vi "Actor Core.vi"(8 "error in":errorcluster, 11 "Settings View in":refnum<class "Settings View.lvclass">) -> (0 "error out":errorcluster={"status"=TRUE, "code"=1556, "source"="In Place Element Structure in Actor Framework.lvlib:Message Priority Queue.lvclass:Priority Enqueue.vi:2960001->Actor Framework MVC.lvlib:Abstract View.lvlib:Abstract View.lvclass:Actor Core.vi:5880008->Settings View.lvlib:Settings View.lvclass:Actor Core.vi"}, 3 "Actor out":refnum<class "Actor.lvclass">)   [LabVIEW 2020, in "Settings View.lvlib" / "Settings View.lvclass"]
doc: "(<B>Filename</B>: Actor Framework.lvlib:Actor.lvclass:Actor Core.vi)\n\nReceives messages to the actor, reacts to them, and initiates any error handling that may shut the actor down.\n\nDescendant classes may override this VI to append parallel tasks for the actor to complete while it handles messages. Overrides use the Call Parent Method node."
uses:
  Settings View.lvclass
  C:/Program Files/National Instruments/LabVIEW 2020/vi.lib/ActorFramework/Actor/Actor.lvclass
  <vilib>/ActorFramework/Actor/Actor.lvclass
  <vilib>/ActorFramework/Actor/Actor.lvclass/Actor.ctl
  <vilib>/ActorFramework/Message Enqueuer/Message Enqueuer.lvclass/Message Enqueuer.ctl
  Settings View Messages/Broadcast Show Grid Msg/Broadcast Show Grid Msg.lvclass/Broadcast Show Grid Msg.ctl
  Settings View Messages/Broadcast Show Origin Msg/Broadcast Show Origin Msg.lvclass/Broadcast Show Origin Msg.ctl
  Settings View Messages/Broadcast Show Tool Label Msg/Broadcast Show Tool Label Msg.lvclass/Broadcast Show Tool Label Msg.ctl
  Settings View Messages/Broadcast Brush Width Msg/Broadcast Brush Width Msg.lvclass/Broadcast Brush Width Msg.ctl
  Settings View Messages/Broadcast Color Table Msg/Broadcast Color Table Msg.lvclass/Broadcast Color Table Msg.ctl
  <vilib>/ActorFramework/Message Enqueuer/Init from Existing Queue.vi
  <vilib>/ActorFramework/Message Enqueuer/Enqueue.vi
  Settings View Messages/Broadcast Show Grid Msg/Broadcast Show Grid Msg.lvclass
  C:/Program Files/National Instruments/LabVIEW 2020/vi.lib/ActorFramework/Message/Message.lvclass
  Settings View Messages/Broadcast Show Origin Msg/Broadcast Show Origin Msg.lvclass
  Settings View Messages/Broadcast Show Tool Label Msg/Broadcast Show Tool Label Msg.lvclass
  Settings View Messages/Broadcast Brush Width Msg/Broadcast Brush Width Msg.lvclass
  Settings View Messages/Broadcast Color Table Msg/Broadcast Color Table Msg.lvclass
  Controllers/UI Controller/UI Controller Messages/Initialize Main View Msg/Initialize Main View Msg.lvclass
  Controllers/UI Controller/UI Controller Messages/Update Occupied Area Msg/Update Occupied Area Msg.lvclass
  <vilib>/ActorFramework/Message Priority Queue/Priority Enqueue.vi
  <vilib>/ActorFrameworkMVC/Abstract View/Abstract View/Abstract View.lvclass
  <vilib>/ActorFramework/Message Enqueuer/Message Enqueuer.lvclass
panel:
  in  "Color Table":T1={"Occupied Color"={"Value"=0, "Color"=0}, "Free Color"={"Value"=254, "Color"=13421772}, "Unknown Color"={"Value"=205, "Color"=16777215}}
  in  "Set Button":bool
  in  "Brush Width Slider":i32(slide)=3 scale=1.0..10.0
  in  "Show Tool Label Button":bool=TRUE
  in  "Show Origin Button":bool
  in  "Show Grid Button":bool
  # "Show grid"
  # "Show origin"
  # "Show tool label"
  # "Brush width"
  # "Occupied color"
  # "Free color"
  # "Unknown color"
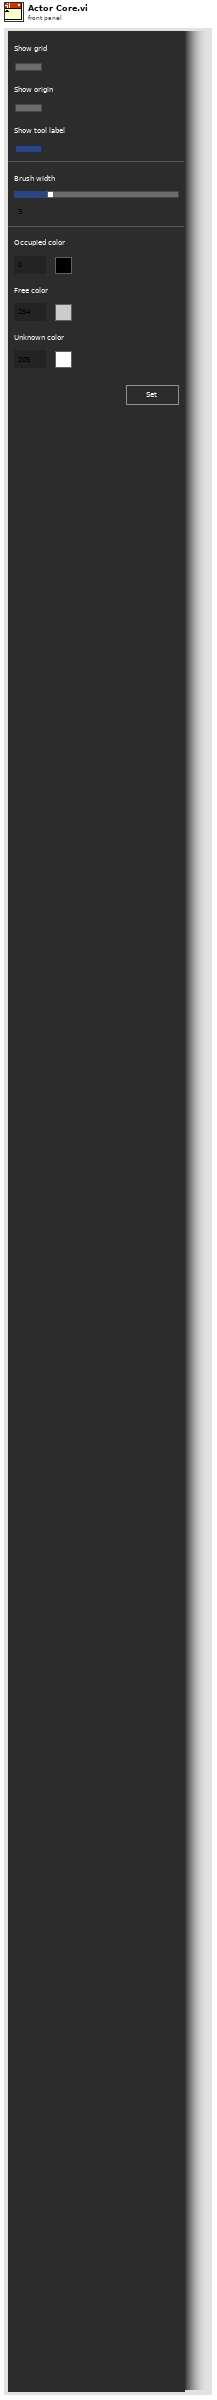
[diagram p1: front panel]
types:
  T1 = cluster{"Occupied Color":cluster{"Value":u8, "Color":u32}, "Free Color":cluster{"Value":u8, "Color":u32}, "Unknown Color":cluster{"Value":u8, "Color":u32}}
  T2 = enum8{"Enabled", "Disabled", "Disabled and Grayed Out"}
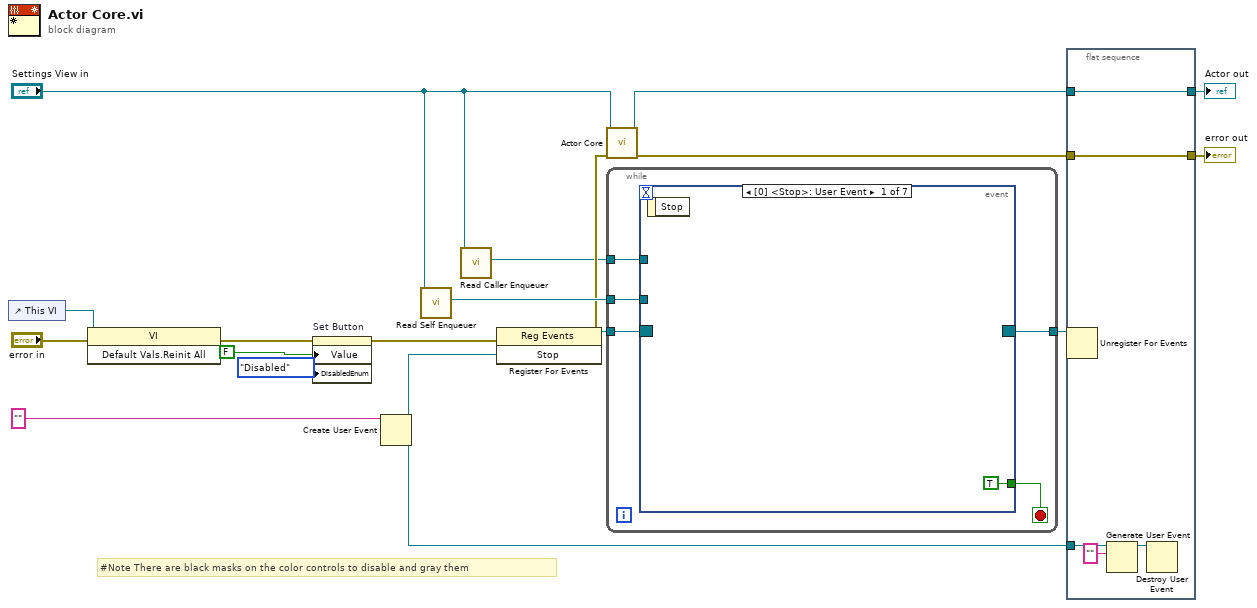
[diagram p0: block diagram]
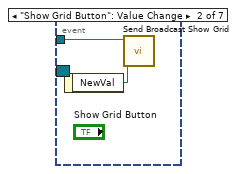
[diagram p2: hidden frame]
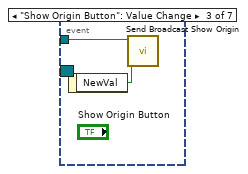
[diagram p3: hidden frame]
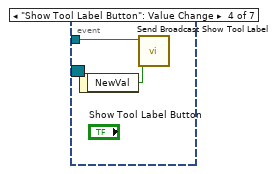
[diagram p4: hidden frame]
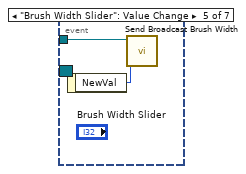
[diagram p5: hidden frame]
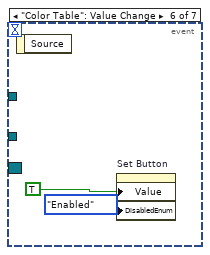
[diagram p6: hidden frame]
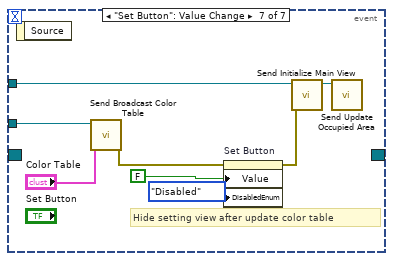
[diagram p7: hidden frame]
diagram:
  # "#Note There are black masks on the color controls to disable and gray them"
  n1 = control-ref of="This VI"() -> (w3:refnum<vi>)
  n2 = invoke class="VI" method="Default Vals.Reinit All"(reference=w3, error in="error in") -> (error out=w4:errorcluster)  [unwired: 1 in, 2 out]
  n3 = property on="Set Button" class="Bool (strict)"(error in=w4, "Value"=FALSE ("Update Button"), "DisabledEnum"=T2."Disabled" ("Disabled")) -> (error out=w5:errorcluster)  [unwired: 1 in, 1 out]
  n4 = Create User Event(user event datatype="" ("Stop")) -> (user event=w12:refnum<user-event>)  [unwired: 1 in, 1 out]
  n5 = call <vilib>:"Read Self Enqueuer.vi"("Actor"="Settings View in") -> ("Self Enqueuer"=w13:refnum<class "Message Enqueuer.lvclass">)  [unwired: 10 in]
  n6 = call <vilib>:"Read Caller Enqueuer.vi"("Actor"="Settings View in") -> ("Caller Enqueuer"=w2:refnum<class "Message Enqueuer.lvclass">)  [unwired: 10 in]
  n7 = register-events(error in=w5, w12) -> (reference out=w16:refnum<event-registration>, error out=w11:errorcluster)  [unwired: 1 in]
  n8 = call-parent "Actor Core.vi"("error in"=w11, "Abstract View in"="Settings View in") -> ("error out"=w14:errorcluster, "Actor out"=w15:refnum<class "Actor.lvclass">)  [unwired: 8 in]
  n9 = while {
    tunnel: w16 -> [w23]
    tunnel: [w22] -> w17
    tunnel: w13 -> [w20]
    tunnel: w2 -> [w19]
    stop <- w21 stop-if-true
    n10 = event shown="[0] <Stop>: User Event" {
      selector: w23 -> [_ _ _ _ _ _ _]
      dyn-events: [_ _ _ _ _ _ _] -> w22
      timeout: _ -> [_ _ _ _ _ _ _]
      tunnel: [TRUE _ _ _ _ _ _] -> w21
      tunnel: w20 -> [_ w26 w28 w30 w32 _ w42]
      tunnel: w19 -> [_ _ _ _ _ _ w36]
      event User Event {
        n11 = event-data() -> ()  [unwired: 1 in, 1 out]
      }
      event "Show Grid Button": Value Change {
        n12 = event-data() -> ("NewVal"=w25:bool)  [unwired: 1 in]
        n13 = call "Send Broadcast Show Grid.vi"("Show Grid"=w25, "Message Enqueuer"=w26) -> ()  [unwired: 8 in, 2 out]
      }
      event "Show Origin Button": Value Change {
        n14 = event-data() -> ("NewVal"=w27:bool)  [unwired: 1 in]
        n15 = call "Send Broadcast Show Origin.vi"("Show Origin"=w27, "Message Enqueuer"=w28) -> ()  [unwired: 8 in, 2 out]
      }
      event "Show Tool Label Button": Value Change {
        n16 = event-data() -> ("NewVal"=w29:bool)  [unwired: 1 in]
        n17 = call "Send Broadcast Show Tool Label.vi"("Show Tool Label"=w29, "Message Enqueuer"=w30) -> ()  [unwired: 8 in, 2 out]
      }
      event "Brush Width Slider": Value Change {
        n18 = event-data() -> ("NewVal"=w31:i32)  [unwired: 1 in]
        n19 = call "Send Broadcast Brush Width.vi"("Brush Width"=w31, "Message Enqueuer"=w32) -> ()  [unwired: 8 in, 2 out]
      }
      event "Color Table": Value Change {
        n20 = event-data() -> ()  [unwired: 1 in, 1 out]
        n21 = property on="Set Button" class="Bool (strict)"("Value"=TRUE ("Update Button"), "DisabledEnum"=T2."Enabled" ("Disabled")) -> ()  [unwired: 2 in, 2 out]
      }
      event "Set Button": Value Change {
        # "Hide setting view after update color table"
        n22 = event-data() -> ()  [unwired: 1 in, 1 out]
        n23 = call "Send Broadcast Color Table.vi"("Color Table"="Color Table", "Message Enqueuer"=w42) -> ("error out"=w38:errorcluster)  [unwired: 8 in, 1 out]
        n24 = property on="Set Button" class="Bool (strict)"(error in=w38, "Value"=FALSE ("Update Button"), "DisabledEnum"=T2."Disabled" ("Disabled")) -> (error out=w35:errorcluster)  [unwired: 1 in, 1 out]
        n25 = call "Send Initialize Main View.vi"("error in (no error)"=w35, "Message Enqueuer"=w36) -> ("Message Enqueuer out"=w37:refnum<class "Message Enqueuer.lvclass">)  [unwired: 8 in, 1 out]
        n26 = call "Send Update Occupied Area.vi"("Message Enqueuer"=w37) -> ()  [unwired: 9 in, 2 out]
      }
    }
  }
  n27 = flat-sequence {
    tunnel: w12 -> [w46]
    tunnel: w15 -> [w44]
    tunnel: [w44] -> w10
    tunnel: [w43] -> w9
    tunnel: w14 -> [w43]
    frame #0 {
      n28 = Generate User Event(user event=w46, event data cluster="" ("event data")) -> (user event out=w47:refnum<user-event>)  [unwired: 2 in, 1 out]
      n29 = Destroy User Event(user event=w47) -> ()  [unwired: 1 in, 1 out]
    }
  }
  n30 = Unregister For Events(event registration refnum=w17) -> ()  [unwired: 1 in, 1 out]
  "error out" <- w9
  "Actor out" <- w10
